vi "BRig_FPGA_v3,94.vi"() -> ()   [LabVIEW 2014]
uses:
  <vilib>/rvi/Emulation/niFpgaGetClockAttributes.vi
  <vilib>/rvi/Emulation/niFpgaSctlEmulationGetInTimedLoop.vi
  <vilib>/rvi/Emulation/niFpgaEmulationReportErrorSimple.vi
  <vilib>/rvi/eio/common/nirviEmuTemplateMethod_errors.vi
  <vilib>/rvi/Emulation/niFpgaCriticalErrorInLSC.vi
  <vilib>/eio/EIONode/EIONode.xnode
panel:
  in  "AnaOut1_Pair":u16
  in  "AnaOut0_Pair":u16
  out "fpga_solenoid_R":bool
  out "fpga_solenoid_L":bool
  out "fpga_laser2":bool
  out "fpga_laser1":bool
  in  "L2Led_ON":bool
  in  "L1Led_ON":bool
  in  "Rising(F)_or_Falling(T)":bool
  in  "Solenoid_trig_R":bool
  in  "Solenoid_trig_L":bool
  in  "Solenoid_nTotal_R":u32=100
  in  "Solenoid_nTotal_L":u32=100
  in  "L2Led_Baseline":bool
  in  "L1Led_Baseline":bool
  in  "CueLed_Baseline":bool
  in  "I_allReward":bool
  in  "AnaOut_1":u16
  in  "CueLed_Event":bool
  in  "CueLed_nValley":u32=100
  in  "CueLed_nPeak":u32=100
  in  "LC_Event_l2":bool
  in  "LC_Laser_l2":bool
  in  "LC_nShutter_l2":u32=100
  in  "LC_nValley_l2":u32=100
  in  "LC_nPeak_l2":u32=100
  in  "LR_wrong_nDelay_l2":u32
  in  "LR_reward_nDelay_l2":u32
  in  "LR_wrong_nTotal_l2":u32=100
  in  "LR_reward_nTotal_l2":u32=100
  in  "LR_wrong_laser_l2":bool
  in  "LR_wrong_Event_l2":bool
  in  "LR_reward_Laser_l2":bool
  in  "LR_reward_Event_l2":bool
  out "AnaIn_1":u16
  out "AnaIn_0":u16
  out "timeTrial_count":u32
  in  "timeTrial_trig":bool
  in  "k1__counter_per_ms":u16=100 min=100 max=40000 step=1
  in  "LC_nShutter_l1":u32=100
  in  "AnaOut_0":u16
  in  "LC_nValley_l1":u32=100
  in  "LC_nPeak_l1":u32=100
  in  "LC_Event_l1":bool
  in  "LR_wrong_nTotal_l1":u32=100
  in  "LR_wrong_nDelay_l1":u32
  in  "LR_reward_nTotal_l1":u32=100
  in  "LR_reward_nDelay_l1":u32
  in  "LR_reward_Event_l1":bool
  in  "LR_wrong_Event_l1":bool
  out "SelectWrong":bool
  out "SelectReward":bool
  in  "LR_wrong_Laser_l1":bool
  in  "LR_reward_Laser_l1":bool
  in  "Left(F)_or_Right(T)":bool
  in  "ignoreWrong":bool
  in  "SelectionState":bool
  in  "LC_Laser_l1":bool
  in  "FPGA_Stop":bool
  in  "audioTrigger_L":bool
  in  "audioTrigger_R":bool
  in  "audioFreq_L_kHz":u8=14 min=1 max=14 step=1
  in  "audioAmp_L":u16=1 min=1 max=32767 step=1
  in  "audioFreq_R_kHz":u8=14 min=1 max=14 step=1
  in  "audioAmp_R":u16=1 min=1 max=32767 step=1
  in  "A3_SL":bool
  in  "A1_SR":bool
  in  "Counts_Reset":bool
  out "A4_LickR":u32
  out "A2_LickL":u32
  in  "A6_Act":bool
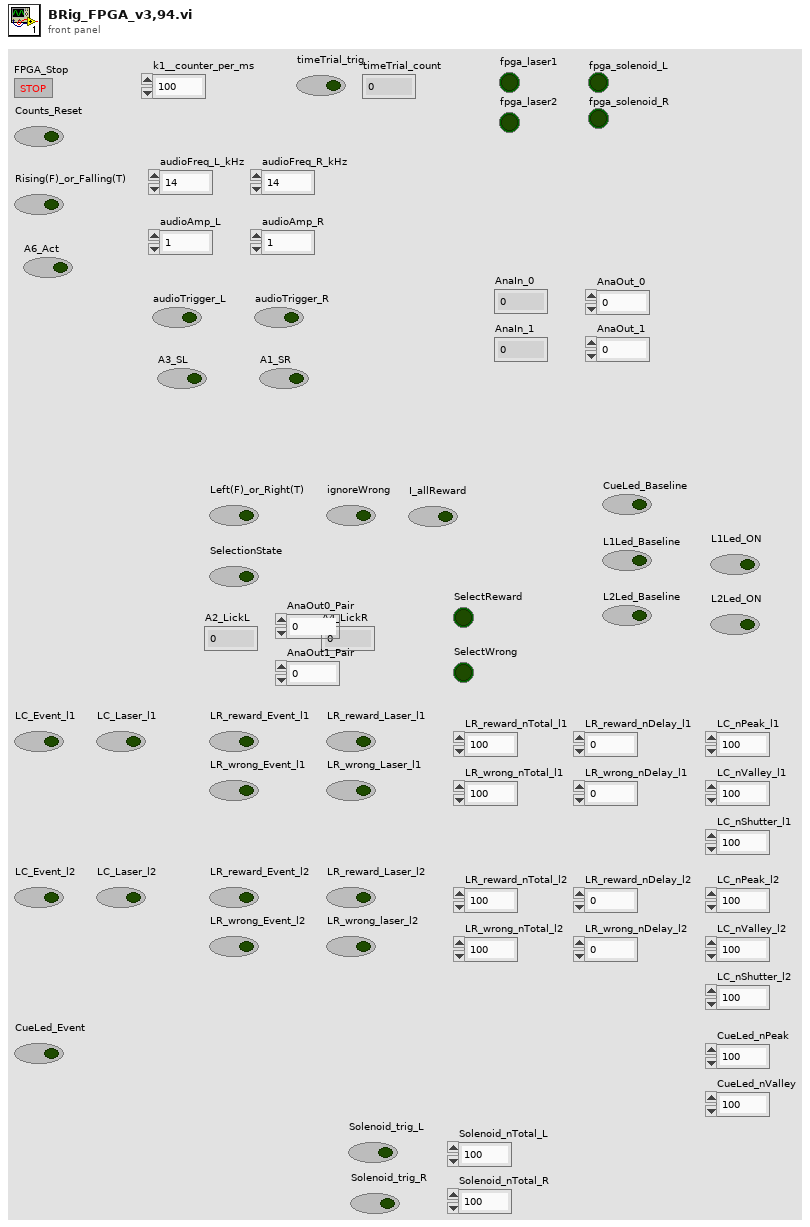
[diagram p1: front panel]
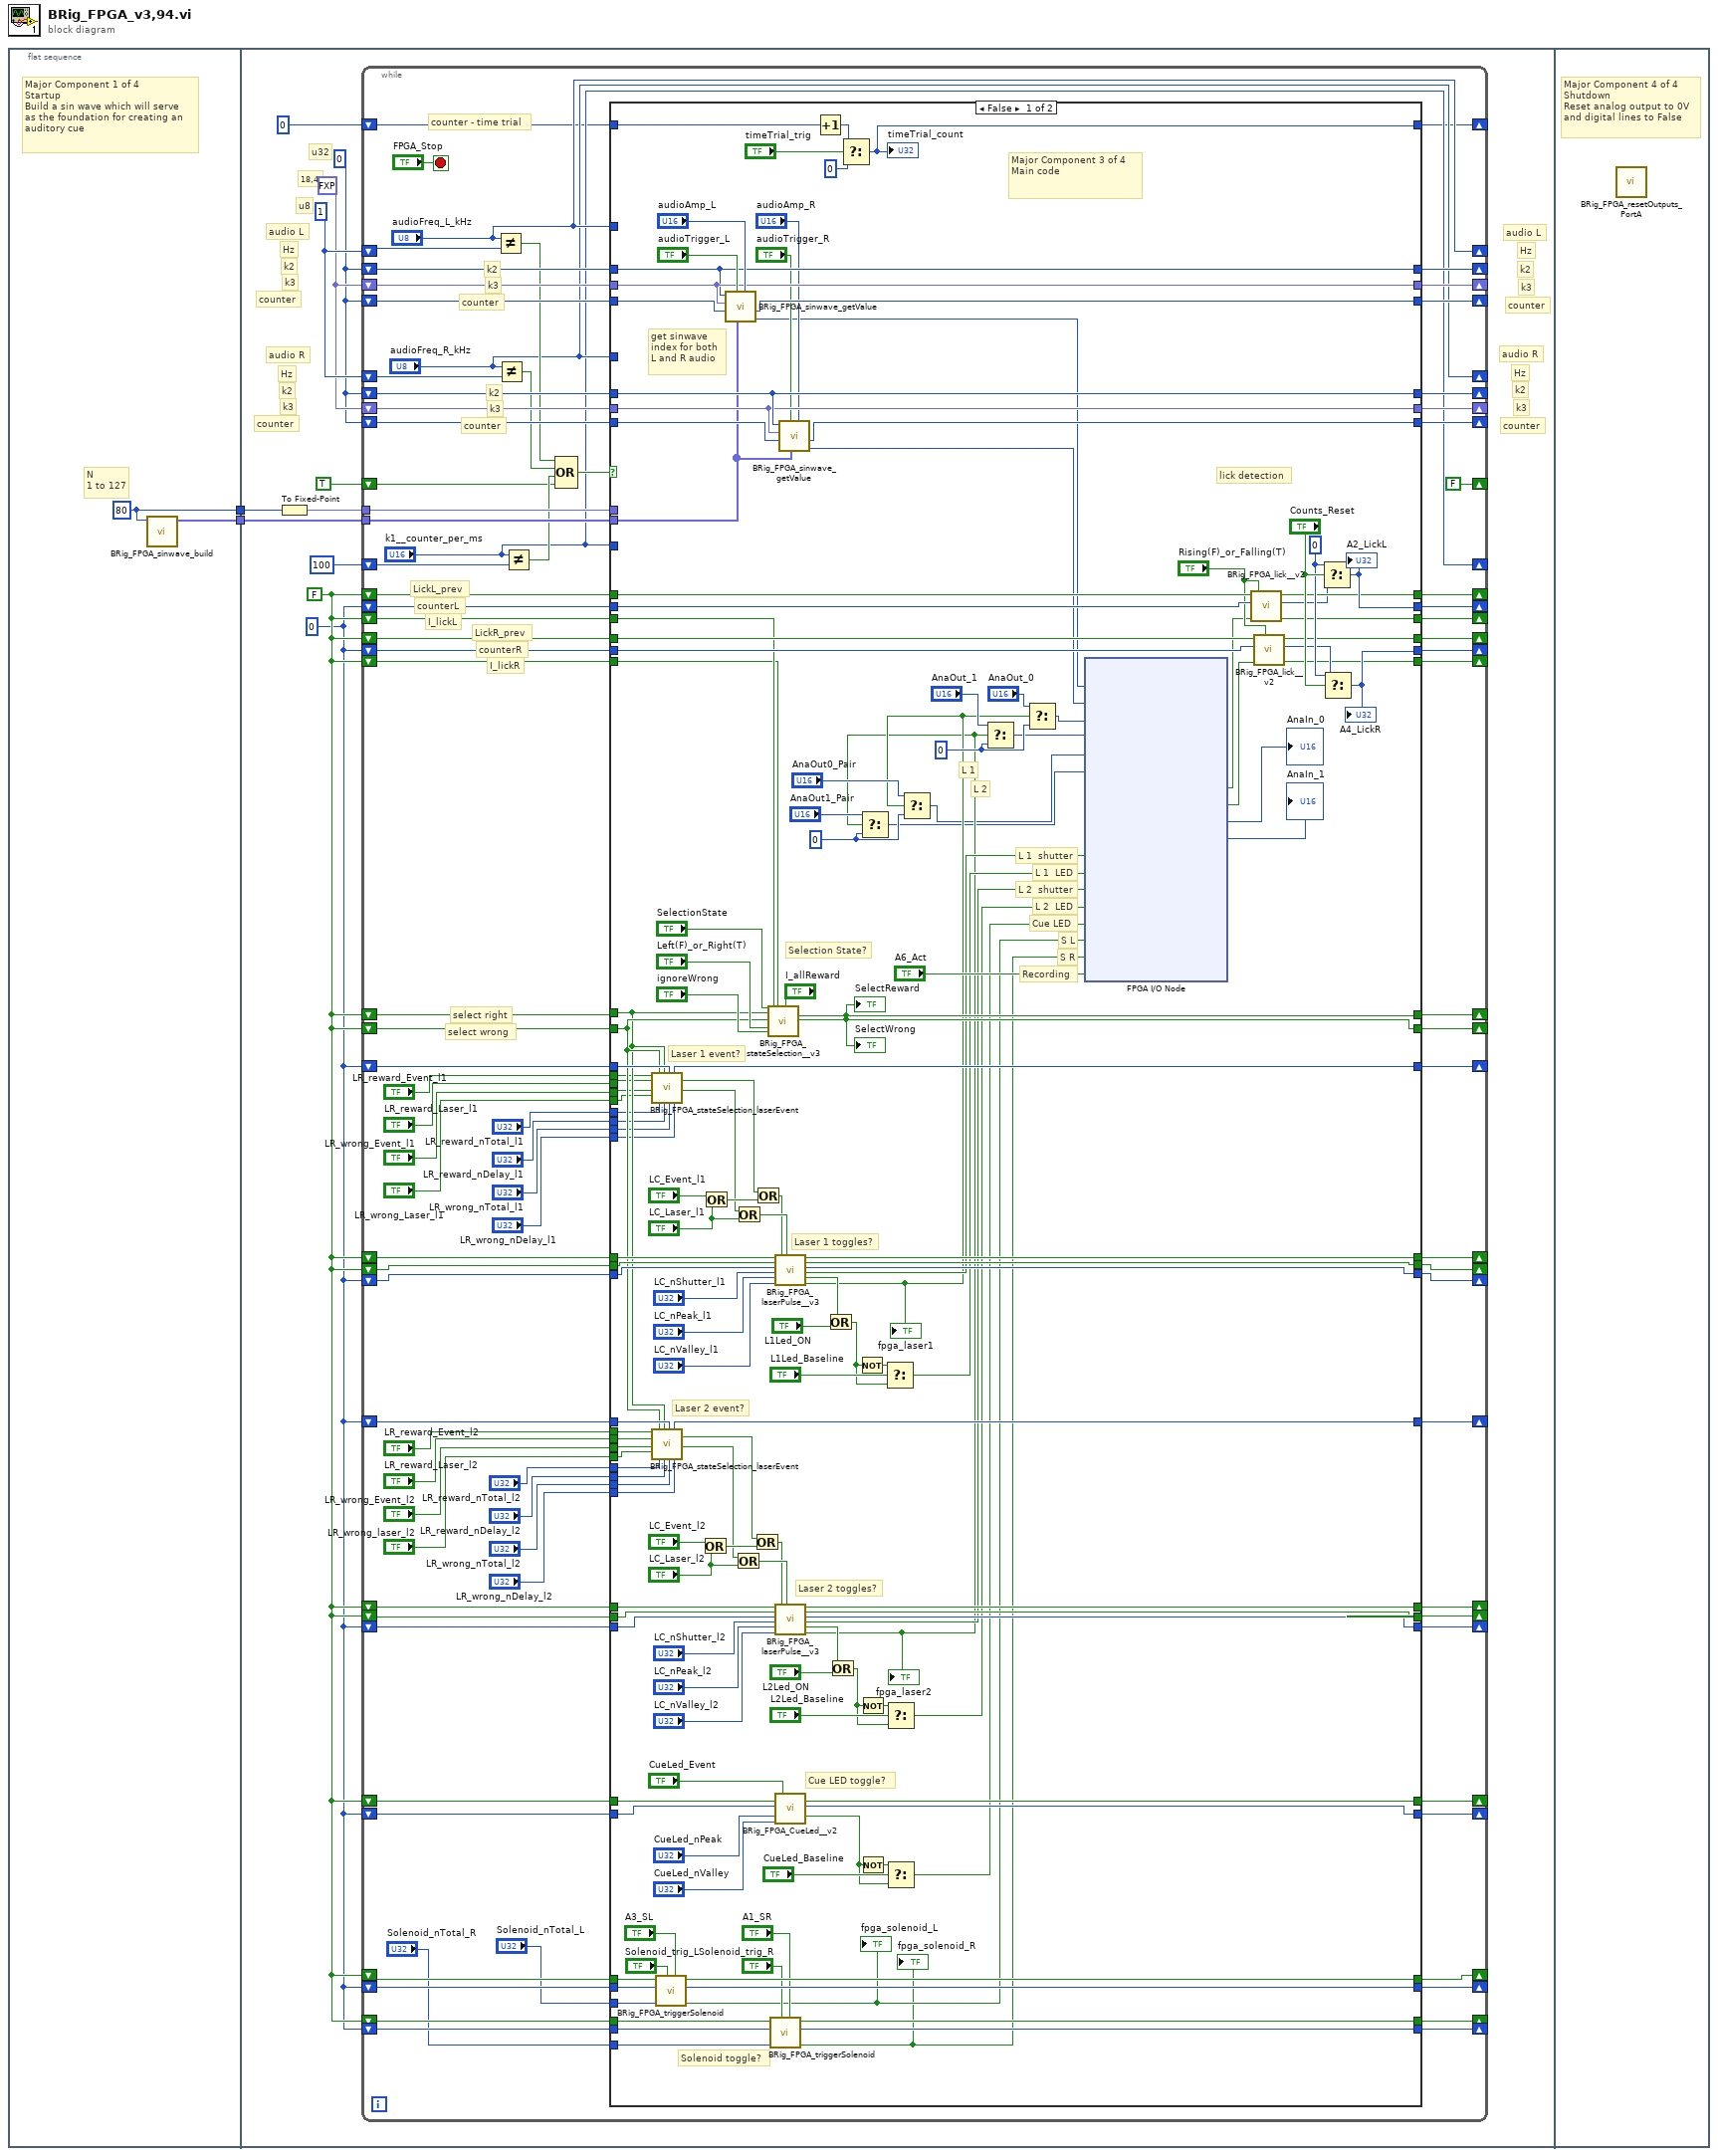
[diagram p0: block diagram]
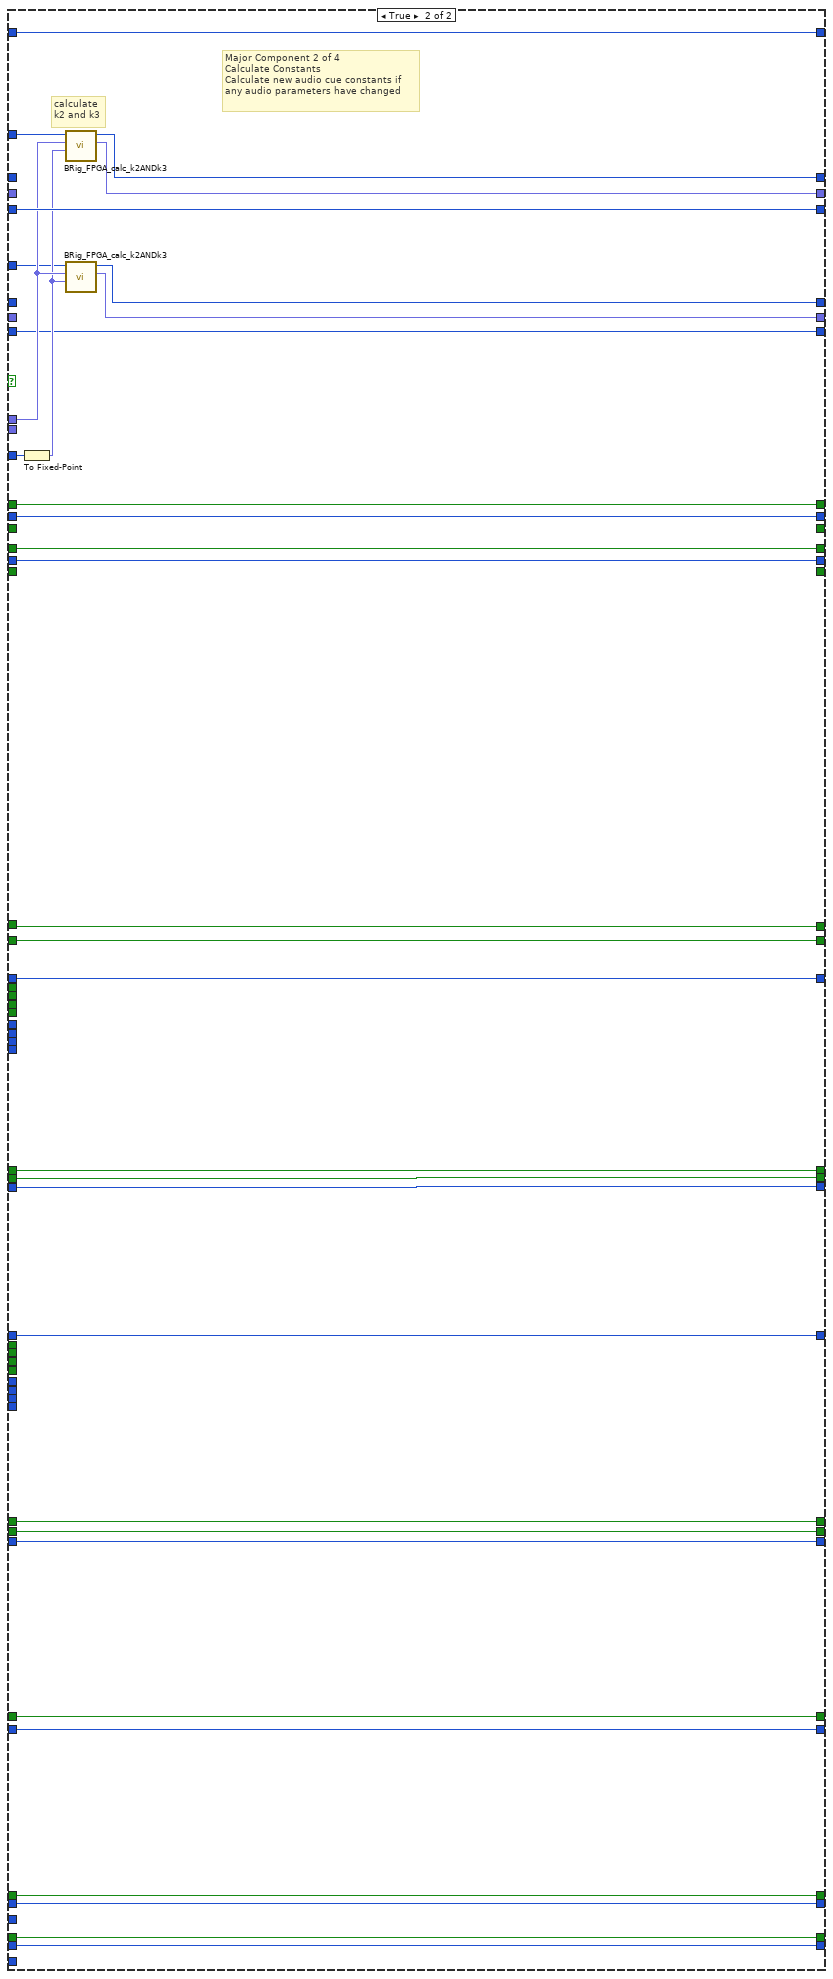
[diagram p2: hidden frame]
diagram:
  n1 = flat-sequence {
    tunnel: [w4] -> w2
    tunnel: [w3] -> w1
    tunnel: w2 -> [w15]
    tunnel: w1 -> [w14]
    frame #0 {
      w3 = 80 ("dimension size")
      # "Major Component 1 of 4\nStartup\nBuild a sin wave which will serve\nas the foundation for creating an\nauditory cue"
      # "N\n1 to 127"
      n2 = call "BRig_FPGA_sinwave_build.vi"("input_Npts"=w3) -> ("output_array_sin"=w4:fxp<+/-,16,2>[])  [unwired: 10 in]
    }
    frame #1 {
      w5 = u32 0
      w6 = FALSE
      w10 = u32 0
      w11 = fxp<+,18,4> 0.0
      w12 = u8 1
      # "counter"
      # "k3"
      # "k2"
      # "counter"
      # "k3"
      # "k2"
      # "counter"
      # "counter"
      # "u32"
      # "k3"
      # "k2"
      # "k3"
      # "18,4"
      # "u8"
      # "Hz"
      # "Hz"
      # "audio R"
      # "audio L"
      # "Hz"
      # "k2"
      # "Hz"
      # "audio R"
      # "audio L"
      n3 = To Fixed-Point(number=w14) -> (fixed-point=w13:fxp<+,7,7>)  [unwired: 1 in]
      n4 = while {
        shift-right: ["audioFreq_L_kHz"] -> _
        shift-left: w12 -> [w106]
        shift-right: [w100] -> _
        shift-left: w10 -> [w104]
        shift-right: ["audioFreq_R_kHz"] -> _
        shift-left: w12 -> [w96]
        tunnel: w15 -> [w103]
        tunnel: w13 -> [w102]
        shift-right: [w99] -> _
        shift-left: w11 -> [w101]
        shift-right: [w97] -> _
        shift-left: w10 -> [w98]
        shift-right: [w94] -> _
        shift-left: w10 -> [w95]
        shift-right: [w92] -> _
        shift-left: w11 -> [w93]
        shift-right: [w90] -> _
        shift-left: w10 -> [w91]
        shift-right: ["k1__counter_per_ms"] -> _
        shift-left: u16 100 ("y") -> [w89]
        shift-right: [FALSE] -> _
        shift-left: TRUE -> [w84]
        shift-right: [w77] -> _
        shift-left: w6 -> [w79]
        shift-right: [w76] -> _
        shift-left: w6 -> [w78]
        shift-right: [w74] -> _
        shift-left: w5 -> [w75]
        shift-right: [w72] -> _
        shift-left: w5 -> [w73]
        shift-right: [w69] -> _
        shift-left: w6 -> [w71]
        shift-right: [w68] -> _
        shift-left: w6 -> [w70]
        shift-right: [w66] -> _
        shift-left: w6 -> [w67]
        shift-right: [w64] -> _
        shift-left: w6 -> [w65]
        shift-right: [w62] -> _
        shift-left: u32 0 -> [w63]
        shift-right: [w60] -> _
        shift-left: w5 -> [w61]
        shift-right: [w59] -> _
        shift-left: w6 -> [w56]
        shift-right: [w58] -> _
        shift-left: w6 -> [w55]
        shift-right: [w57] -> _
        shift-left: w5 -> [w54]
        shift-right: [w52] -> _
        shift-left: w5 -> [w53]
        shift-right: [w51] -> _
        shift-left: w6 -> [w48]
        shift-right: [w50] -> _
        shift-left: w6 -> [w47]
        shift-right: [w49] -> _
        shift-left: w5 -> [w46]
        shift-right: [w45] -> _
        shift-left: w6 -> [w43]
        shift-right: [w44] -> _
        shift-left: w5 -> [w42]
        shift-right: [w24] -> _
        shift-left: w5 -> [w25]
        shift-right: [w21] -> _
        shift-left: w6 -> [w23]
        shift-right: [w18] -> _
        shift-left: w6 -> [w20]
        shift-right: [w17] -> _
        shift-left: w5 -> [w19]
        stop <- "FPGA_Stop" stop-if-true
        # "counter"
        # "k3"
        # "k2"
        # "counter"
        # "k3"
        # "k2"
        # "counter - time trial"
        # "I_lickR"
        # "counterR"
        # "LickR_prev"
        # "I_lickL"
        # "counterL"
        # "LickL_prev"
        # "select wrong"
        # "select right"
        n5 = Not Equal?(x="audioFreq_L_kHz", y=w106) -> (x != y?=w88:bool)
        n6 = Not Equal?(x="audioFreq_R_kHz", y=w96) -> (x != y?=w87:bool)
        n7 = Not Equal?(x="k1__counter_per_ms", y=w89) -> (x != y?=w85:bool)
        n8 = Compound Arithmetic op=OR(w88, w87, w85, w84) -> (w86:bool)
        n9 = case shown="False" w86 {
          tunnel: w104 -> [w246 _]
          tunnel: "audioFreq_L_kHz" -> [_ w292]
          tunnel: w103 -> [w239 _]
          tunnel: w102 -> [_ w288]
          tunnel: "k1__counter_per_ms" -> [_ w293]
          tunnel: w101 -> [w247 _]
          tunnel: [w246 w291] -> w100
          tunnel: [w247 w290] -> w99
          tunnel: w98 -> [w251 w289]
          tunnel: [w248 w289] -> w97
          tunnel: w95 -> [w243 _]
          tunnel: [w243 w284] -> w94
          tunnel: w93 -> [w242 _]
          tunnel: [w242 w285] -> w92
          tunnel: w91 -> [w245 w283]
          tunnel: "audioFreq_R_kHz" -> [_ w286]
          tunnel: [w244 w283] -> w90
          tunnel: w79 -> [w234 w282]
          tunnel: w78 -> [w233 w281]
          tunnel: [w238 w282] -> w77
          tunnel: [w231 w281] -> w76
          tunnel: w75 -> [w235 w280]
          tunnel: [w261 w280] -> w74
          tunnel: w73 -> [w232 w279]
          tunnel: [w258 w279] -> w72
          tunnel: w71 -> [w189 w278]
          tunnel: w70 -> [w190 w277]
          tunnel: [w209 w278] -> w69
          tunnel: [w254 w277] -> w68
          tunnel: [w224 w274] -> w59
          tunnel: [w225 w273] -> w58
          tunnel: [w226 w272] -> w57
          tunnel: w67 -> [w228 _]
          tunnel: [w237 _] -> w66
          tunnel: w65 -> [w227 _]
          tunnel: [w229 _] -> w64
          tunnel: w63 -> [w216 w276]
          tunnel: [w213 w276] -> w62
          tunnel: w61 -> [w208 w275]
          tunnel: [w207 w275] -> w60
          tunnel: w56 -> [w206 w274]
          tunnel: w55 -> [w205 w273]
          tunnel: w54 -> [w204 w272]
          tunnel: w53 -> [w192 w271]
          tunnel: [w191 w271] -> w52
          tunnel: [w187 w270] -> w51
          tunnel: [w186 w269] -> w50
          tunnel: [w185 w268] -> w49
          tunnel: w48 -> [w184 w270]
          tunnel: w47 -> [w183 w269]
          tunnel: w46 -> [w182 w268]
          tunnel: [w179 w267] -> w45
          tunnel: [w178 w266] -> w44
          tunnel: w43 -> [w177 w267]
          tunnel: w42 -> [w176 w266]
          tunnel: "LR_reward_Event_l1" -> [w162 _]
          tunnel: "LR_reward_Laser_l1" -> [w161 _]
          tunnel: "LR_wrong_Event_l1" -> [w160 _]
          tunnel: "LR_wrong_Laser_l1" -> [w159 _]
          tunnel: "LR_reward_nTotal_l1" -> [w158 _]
          tunnel: "LR_reward_nDelay_l1" -> [w157 _]
          tunnel: "LR_wrong_nTotal_l1" -> [w156 _]
          tunnel: "LR_wrong_nDelay_l1" -> [w155 _]
          tunnel: "LR_reward_Event_l2" -> [w154 _]
          tunnel: "LR_reward_Laser_l2" -> [w153 _]
          tunnel: "LR_wrong_Event_l2" -> [w152 _]
          tunnel: "LR_wrong_laser_l2" -> [w151 _]
          tunnel: "LR_reward_nTotal_l2" -> [w150 _]
          tunnel: "LR_reward_nDelay_l2" -> [w149 _]
          tunnel: "LR_wrong_nTotal_l2" -> [w148 _]
          tunnel: "LR_wrong_nDelay_l2" -> [w147 _]
          tunnel: w25 -> [w146 w265]
          tunnel: [w141 w265] -> w24
          tunnel: w23 -> [w145 w264]
          tunnel: "Solenoid_nTotal_L" -> [w144 _]
          tunnel: [w140 w264] -> w21
          tunnel: w20 -> [w137 w263]
          tunnel: w19 -> [w136 w262]
          tunnel: [w135 w263] -> w18
          tunnel: [w134 w262] -> w17
          tunnel: "Solenoid_nTotal_R" -> [w133 _]
          frame False {
            w112 = u16 0 ("f")
            w173 = u16 0 ("f")
            w259 = u32 0 ("t")
            # "Cue LED"
            # "L 2  shutter"
            # "L 2  LED"
            # "L 1  shutter"
            # "L 1  LED"
            # "Recording"
            # "S L"
            # "S R"
            # "L 2"
            # "L 1"
            # "Solenoid toggle?"
            # "Cue LED toggle?"
            # "Laser 2 toggles?"
            # "Laser 2 event?"
            # "Laser 1 toggles?"
            # "Selection State?"
            # "Laser 1 event?"
            # "Major Component 3 of 4\nMain code"
            # "get sinwave\nindex for both\nL and R audio"
            # "lick detection"
            n10 = call "BRig_FPGA_stateSelection_laserEvent.vi"("I_LR_reward"=w162, "I_LR_reward_laser"=w161, "I_LR_wrong"=w160, "I_LR_wrong_laser"=w159, "I_selectWrong"=w190, "laser_reward_nTotal"=w158, "I_selectReward"=w189, "laser_reward_nDelay"=w157, "counter"=w208, "laser_wrong_nTotal"=w156, "laser_wrong_nDelay"=w155) -> ("output_counter"=w207:u32, "output_I_laserEvent"=w203:bool, "output_I_laserOn"=w202:bool)  [unwired: 6 in]
            n11 = call "BRig_FPGA_stateSelection_laserEvent.vi"("I_LR_reward"=w154, "I_LR_reward_laser"=w153, "I_LR_wrong"=w152, "I_LR_wrong_laser"=w151, "I_selectWrong"=w190, "laser_reward_nTotal"=w150, "I_selectReward"=w189, "laser_reward_nDelay"=w149, "counter"=w192, "laser_wrong_nTotal"=w148, "laser_wrong_nDelay"=w147) -> ("output_counter"=w191:u32, "output_I_laserEvent"=w188:bool, "output_I_laserOn"=w193:bool)  [unwired: 6 in]
            n12 = call "BRig_FPGA_triggerSolenoid.vi"("input_Solenoid_MTrig"="A3_SL", "input_Solenoid_trig"="Solenoid_trig_L", "input_threshold"=w144, "input_counter"=w146, "input_trig"=w145) -> ("output_Solenoid_OnOff"=w115:bool, "output_counter"=w141:u32, "output_trig"=w140:bool)  [unwired: 4 in]
            "fpga_solenoid_L" <- w115
            n13 = Or(x="LC_Event_l2", y="LC_Laser_l2") -> (x .or. y?=w197:bool)
            n14 = Or(x="LC_Event_l1", y="LC_Laser_l1") -> (x .or. y?=w220:bool)
            n15 = call "BRig_FPGA_sinwave_getValue.vi"("audioAmp"="audioAmp_L", "sinwave"=w239, "audioTrigger"="audioTrigger_L", "counter"=w251, "k3"=w247, "k2"=w246) -> ("output_audioValue"=w211:i16, "output_counter"=w248:u32)  [unwired: 4 in]
            n16 = Or(x=w193, y="LC_Laser_l2") -> (x .or. y?=w195:bool)
            n17 = Or(x=w202, y="LC_Laser_l1") -> (x .or. y?=w218:bool)
            n18 = Or(x=w188, y=w197) -> (x .or. y?=w194:bool)
            n19 = Or(x=w203, y=w220) -> (x .or. y?=w217:bool)
            n20 = call "BRig_FPGA_stateSelection__v3.vi"("I_selectionState"="SelectionState", "I_selectRight"=w189, "I_selectWrong"=w190, "I_Left(F)_or_Right(T)"="Left(F)_or_Right(T)", "I_ignoreWrong"="ignoreWrong", "I_lickL"=w228, "I_lickR"=w227, "I_allReward"="I_allReward") -> ("output__I_selectRight"=w209:bool, "output__I_selectWrong"=w254:bool)  [unwired: 18 in]
            "SelectWrong" <- w254
            "SelectReward" <- w209
            n21 = call "BRig_FPGA_triggerSolenoid.vi"("input_Solenoid_MTrig"="A1_SR", "input_Solenoid_trig"="Solenoid_trig_R", "input_threshold"=w133, "input_counter"=w136, "input_trig"=w137) -> ("output_Solenoid_OnOff"=w114:bool, "output_counter"=w134:u32, "output_trig"=w135:bool)  [unwired: 4 in]
            "fpga_solenoid_R" <- w114
            n22 = call "BRig_FPGA_laserPulse__v3.vi"("I_shutter"=w206, "I_peak"=w205, "count"=w204, "laser_Nshutter"="LC_nShutter_l1", "laser_Npeak"="LC_nPeak_l1", "laser_Nvalley"="LC_nValley_l1", "I_laserEvent"=w217, "I_laser"=w218) -> ("output_I_shutter"=w224:bool, "output_I_peak"=w225:bool, "output_count"=w226:u32, "output_shutter"=w120:bool, "output_led"=w130:bool, "output_laser"=w110:bool)  [unwired: 6 in]
            "fpga_laser1" <- w110
            n23 = call "BRig_FPGA_laserPulse__v3.vi"("I_shutter"=w184, "I_peak"=w183, "count"=w182, "laser_Nshutter"="LC_nShutter_l2", "laser_Npeak"="LC_nPeak_l2", "laser_Nvalley"="LC_nValley_l2", "I_laserEvent"=w194, "I_laser"=w195) -> ("output_I_shutter"=w187:bool, "output_I_peak"=w186:bool, "output_count"=w185:u32, "output_shutter"=w118:bool, "output_led"=w127:bool, "output_laser"=w109:bool)  [unwired: 6 in]
            "fpga_laser2" <- w109
            n24 = call "BRig_FPGA_CueLed__v2.vi"("I_peak"=w177, "count"=w176, "laser_Npeak"="CueLed_nPeak", "laser_Nvalley"="CueLed_nValley", "I_CueLed_Event"="CueLed_Event") -> ("output_I_peak"=w179:bool, "output_count"=w178:u32, "output_led"=w167:bool)  [unwired: 12 in]
            n25 = call "BRig_FPGA_sinwave_getValue.vi"("audioAmp"="audioAmp_R", "sinwave"=w239, "audioTrigger"="audioTrigger_R", "counter"=w245, "k3"=w242, "k2"=w243) -> ("output_audioValue"=w210:i16, "output_counter"=w244:u32)  [unwired: 4 in]
            n26 = Increment(x=w216) -> (x+1=w215:u32)
            n27 = Or(x=w130, y="L1Led_ON") -> (x .or. y?=w129:bool)
            n28 = Or(x=w127, y="L2Led_ON") -> (x .or. y?=w126:bool)
            n29 = Select(t=w215, s="timeTrial_trig", f=u32 0) -> (s? t:f=w213:u32)
            "timeTrial_count" <- w213
            n30 = Not(x=w129) -> (.not. x?=w166:bool)
            n31 = Not(x=w126) -> (.not. x?=w164:bool)
            n32 = Not(x=w167) -> (.not. x?=w169:bool)
            n33 = Select(t="AnaOut1_Pair", s=w109, f=w112) -> (s? t:f=w108:u16)
            n34 = Select(t=w166, s="L1Led_Baseline", f=w129) -> (s? t:f=w119:bool)
            n35 = Select(t=w164, s="L2Led_Baseline", f=w126) -> (s? t:f=w117:bool)
            n36 = Select(t=w169, s="CueLed_Baseline", f=w167) -> (s? t:f=w116:bool)
            n37 = Select(t="AnaOut0_Pair", s=w110, f=w112) -> (s? t:f=w107:u16)
            n38 = Select(t="AnaOut_1", s=w109, f=w173) -> (s? t:f=w171:u16)
            n39 = Select(t="AnaOut_0", s=w110, f=w173) -> (s? t:f=w174:u16)
            n40 = xnode "FPGA I/O Node"("AudioOut/Left"=w211, "AudioOut/Right"=w210, "ConnectorB/AO0"=w174, "ConnectorB/AO1"=w171, "ConnectorA/AO0"=w107, "ConnectorA/AO1"=w108, "ConnectorA/DIO6"=w120, "ConnectorB/DIO14"=w119, "ConnectorA/DIO7"=w118, "ConnectorB/DIO15"=w117, "ConnectorB/DIO9"=w116, "ConnectorA/DIO3"=w115, "ConnectorA/DIO5"=w114, "ConnectorA/DIO0"="A6_Act") -> ("ConnectorA/DIO4"=w125:bool, "ConnectorA/DIO2"=w124:bool, "ConnectorB/AI1"=→"AnaIn_0":u16, "ConnectorB/AI2"=→"AnaIn_1":u16)  [unwired: 18 in, 18 out]
            n41 = call "BRig_FPGA_lick__v2.vi"("Rising(F)_or_Falling(T)"="Rising(F)_or_Falling(T)", "I_stateDetector_new"=w125, "counter"=w235, "I_stateDetector_prev"=w234) -> ("output_I_lick"=w237:bool, "output_counter"=w236:u32, "output_I_stateDetector_prev"=w238:bool)  [unwired: 5 in]
            n42 = call "BRig_FPGA_lick__v2.vi"("Rising(F)_or_Falling(T)"="Rising(F)_or_Falling(T)", "I_stateDetector_new"=w124, "counter"=w232, "I_stateDetector_prev"=w233) -> ("output_I_lick"=w229:bool, "output_counter"=w230:u32, "output_I_stateDetector_prev"=w231:bool)  [unwired: 5 in]
            n43 = Select(t=w259, s="Counts_Reset", f=w236) -> (s? t:f=w261:u32)
            "A2_LickL" <- w261
            n44 = Select(t=w259, s="Counts_Reset", f=w230) -> (s? t:f=w258:u32)
            "A4_LickR" <- w258
          }
          frame True {
            # "Major Component 2 of 4\nCalculate Constants\nCalculate new audio cue constants if\nany audio parameters have changed"
            # "calculate\nk2 and k3"
            n45 = To Fixed-Point(number=w293) -> (fixed-point=w287:fxp<+,16,16>)  [unwired: 1 in]
            n46 = call "BRig_FPGA_calc_k2ANDk3.vi"("input_k1[count/ms]"=w287, "input_Npts"=w288, "input_freq[kHz]"=w292) -> ("output_k3"=w290:fxp<+,18,4>, "output_k2"=w291:u32)  [unwired: 7 in]
            n47 = call "BRig_FPGA_calc_k2ANDk3.vi"("input_k1[count/ms]"=w287, "input_Npts"=w288, "input_freq[kHz]"=w286) -> ("output_k3"=w285:fxp<+,18,4>, "output_k2"=w284:u32)  [unwired: 7 in]
          }
        }
      }
    }
    frame #2 {
      # "Major Component 4 of 4\nShutdown\nReset analog output to 0V\nand digital lines to False"
      n48 = call "BRig_FPGA_resetOutputs_PortA.vi"() -> ()  [unwired: 12 in]
    }
  }
